vi "MultiTrigBurst.vi"(2 "high time":dbl=1e-05 format="%^.2e", 3 "Digitizer Settings":T1={"Digitizer delay (us) "=0.0, "rf points per line"=2048, "lines per plane"=128, "Samp Rate (Hz)"=100000000.0, "Additional dig delay (us)"=0.0, "Voltage Scale"=0.4, "Pre-Looks"=0, "Offset delay (us)"=0.0, "bits A/D"=8, "Avg Num"=1, "DigTimeOut"=5.0, "Rel Dig Delay"=0.0, "Dig Ch"=0, "LeCroyCluster"={"LeCroy Channels"=[TRUE, FALSE, FALSE, FALSE], "LC read pt offset"=0.0, "Sweep Avg"=FALSE}, "Main Digitizer"=enum."NI Digitizer", "Dig Config"=enum."Single channel", "Digitizer ID Cluster"={"Acqiris/Alazar/SP ID"=[], "NI Instr Handles"=[], "LeCroy VISA"="", "GaGe Handle"={"Handle"=0, "Sample size"=0, "Resolution"=0, "Offset"=0, "Channels"=0, "Boards"=0}, "ATS Ref"="ATS9350", "Acqiris Address"=["PCI::INSTR0"], "ADQRef"=refnum, "adq_cu_ptr"=refnum}, "Trigger Settings"={"Trig Source"=1, "Trig Coupling"=0, "Trig Slope"=0, "Level (mV)"=1500.0}, "Bulk Acq"=FALSE, "Bulk Start Indexes"=[], "Data Ref RF"=refnum, "NI ID/Channel"=[], "Total Dig CH"=1, "Xtra Ann Trig delay (us)"=10.0, "Fix Z Delay?"=FALSE, "One Way Transmission?"=FALSE, "Data Ref Log"=refnum} {"Trigger Settings"."Trig Slope" items=["Positive", "Negative"]; "Trigger Settings"."Level (mV)" format="%.2f"; "Trigger Settings"."Trig Coupling" items=["DC 1 MOhm", "AC 1 MOhm", "DC 50 Ohm", "AC 50 Ohm"]; "Trigger Settings"."Trig Source" items=["Chan 1", "External"]; "Rel Dig Delay" format="%.2f"; "DigTimeOut" format="%.2f"; "Avg Num" min=1; "Offset delay (us)" format="%.2f"; "Additional dig delay (us)" format="%.2f"; "Digitizer delay (us)" format="%.2f"}, 4 "error in":errorcluster, 5 "Output Pulse#":i32=2, 6 "Counter(s)":tag="Dev1/ctr1", 7 "Source":tag="/Dev1/PFI9" caption="Trigger Source") -> (0 "error out":errorcluster, 1 "task out":refnum<k21>)   [LabVIEW 2022 SP3]
uses:
  Digitizers/-DigitizerRoutines/DigitizerSettings.ctl
  Digitizers/-DigitizerRoutines/Digitizer.ctl
  Digitizers/-DigitizerRoutines/DigConfig.ctl
  Digitizers/-DigitizerRoutines/DigitizerID.ctl
  C:/Windows/System32/ADQAPI_dotNet_helper.dll
  Motion Controllers/-MotionRoutines/MotionGlobals.vi
  Switch Modules/SwitchGlobals.vi
  <vilib>/DAQmx/create/channels.llb/DAQmx Create Channel (CO-Pulse Generation-Time).vi
  <vilib>/DAQmx/configure/timing.llb/DAQmx Timing (Implicit).vi
  <vilib>/DAQmx/configure/trigger.llb/DAQmx Start Trigger (Digital Edge).vi
  <resource>/objmgr/daqmx.rc
panel:
  in  "Trigger Edge":i32(ring)=10280 items=["Rising"=10280, "Falling"=10171]
  # "Counter 1 output is the BNC on grey box."
  # "Trigger source comes from Gate of CTR0 (PFI9)\n\nThe NI trigger connector routes to CTR0 Gate\n\nConnect Ther Ext Trigger to digitizer\n\nNeed to turn global variable on for Retro pulse\n\nUse delay and window pluse high time to determine interval between"
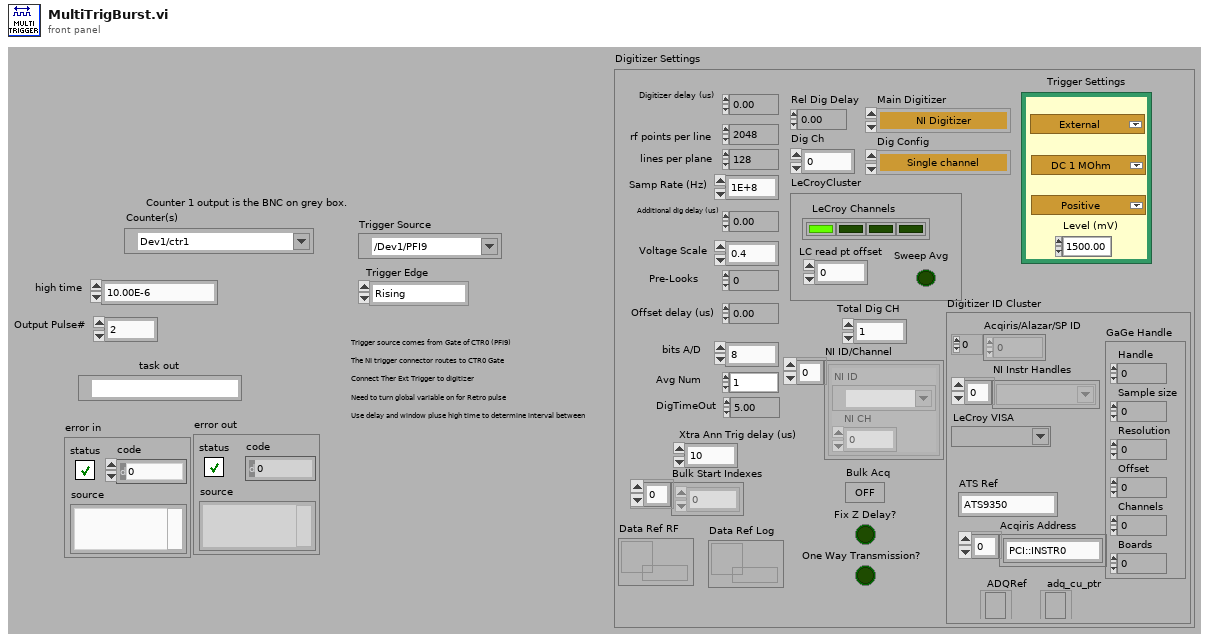
[diagram p1: front panel]
types:
  T1 = typedef "DigitizerSettings.ctl" = cluster{"Digitizer delay (us) ":dbl, "rf points per line":i32, "lines per plane":i32, "Samp Rate (Hz)":dbl, "Additional dig delay (us)":dbl, "Voltage Scale":dbl, "Pre-Looks":i32, "Offset delay (us)":dbl, "bits A/D":i8, "Avg Num":i32, "DigTimeOut":sgl, "Rel Dig Delay":sgl, "Dig Ch":i32, "LeCroyCluster":cluster{"LeCroy Channels":bool[], "LC read pt offset":dbl, "Sweep Avg":bool}, "Main Digitizer":T2, "Dig Config":T3, "Digitizer ID Cluster":T4, "Trigger Settings":cluster{"Trig Source":u16, "Trig Coupling":u16, "Trig Slope":u16, "Level (mV)":dbl}, "Bulk Acq":bool, "Bulk Start Indexes":i32[], "Data Ref RF":refnum<data-value>, "NI ID/Channel":cluster{"NI ID":refnum<k15>, "NI CH":i32}[], "Total Dig CH":i32, "Xtra Ann Trig delay (us)":dbl, "Fix Z Delay?":bool, "One Way Transmission?":bool, "Data Ref Log":refnum<data-value>}
  T2 = typedef "Digitizer.ctl" = enum16{"Acqiris Digitizer", "NI Digitizer", "LeCroy", "GaGe", "AlazarTech", "No Digitizer", "Teledyne"}
  T3 = typedef "DigConfig.ctl" = enum16{"Single channel", "2 Chans w/ 2 Acqiris", "2 Chans w/ 1 Acqiris", "5-CH Pulser New", "5-CH pulser w/ ann array", "5-pass style ann array", "Empty"}
  T4 = typedef "DigitizerID.ctl" = cluster{"Acqiris/Alazar/SP ID":u32[], "NI Instr Handles":refnum<k15>[], "LeCroy VISA":refnum<visa-resource-name>, "GaGe Handle":cluster{"Handle":u32, "Sample size":u32, "Resolution":i32, "Offset":i32, "Channels":u32, "Boards":u32}, "ATS Ref":string, "Acqiris Address":string[], "ADQRef":refnum<k24>, "adq_cu_ptr":refnum<k24>}
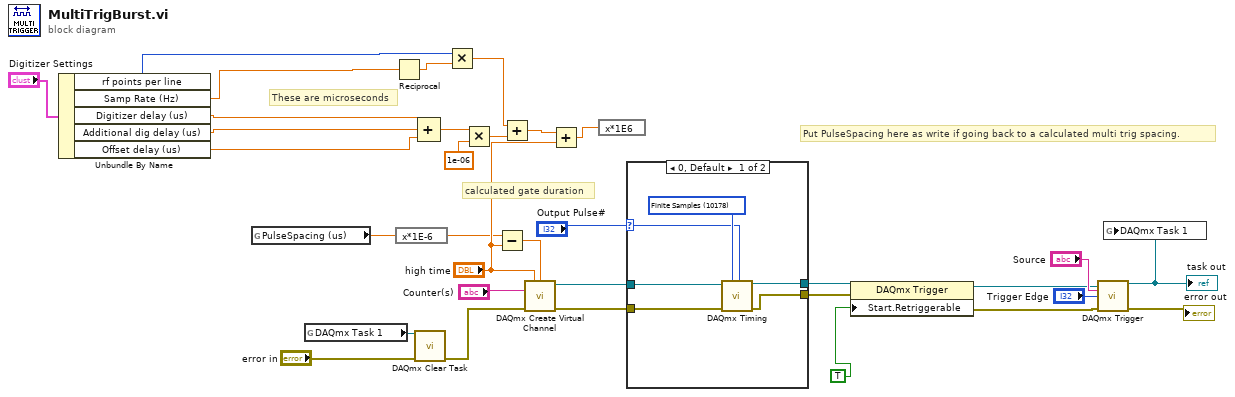
[diagram p0: block diagram]
diagram:
  # "Put PulseSpacing here as write if going back to a calculated multi trig spacing."
  # "calculated gate duration"
  # "These are microseconds"
  n1 = Unbundle By Name("Digitizer Settings") -> ("rf points per line"=w6:i32, "Samp Rate (Hz)"=w7:dbl, "Digitizer delay (us)"=w5:dbl, "Additional dig delay (us)"=w4:dbl, "Offset delay (us)"=w3:dbl)
  n2 = global read "SwitchGlobals.vi" "PulseSpacing (us)"() -> (w1:sgl)
  n3 = global read "MotionGlobals.vi" "DAQmx Task 1"() -> (w16:refnum<k21>)
  n4 = Reciprocal(x=w7) -> (1/x=w18:dbl)
  n5 = expression code="x*1E-6"(w1) -> (w10:sgl)
  n6 = call <vilib>:"DAQmx Clear Task.vi"("task in"=w16, "error in"="error in") -> ("error out"=w15:errorcluster)  [unwired: 13 out]
  n7 = Compound Arithmetic op=ADD(w5, w4, w3) -> (w27:dbl)
  n8 = Multiply(x=w6, y=w18) -> (x*y=w25:dbl)
  n9 = Multiply(x=w27, y=1e-06) -> (x*y=w24:dbl)
  n10 = Subtract(x=w10, y="high time") -> (x-y=w11:dbl)
  n11 = Add(x=w25, y=w24) -> (x+y=w12:dbl)
  n12 = call-poly <vilib>:"DAQmx Create Virtual Channel.vi"("high time"="high time", "low time"=w11, "counter"="Counter(s)", "error in"=w15) -> ("task out"=w32:refnum<k21>, "error out"=w33:errorcluster)  [unwired: 5 in, 5 out]
  n13 = Add(x=w12, y="high time") -> (x+y=w14:dbl)
  n14 = expression code="x*1E6"(w14) -> ()  [unwired: 1 out]
  n15 = case shown="0, Default" "Output Pulse#" {
    selector: "Output Pulse#" -> [w34 _]
    tunnel: w33 -> [w39 w40]
    tunnel: w32 -> [w38 w41]
    tunnel: [w36 w41] -> w23
    tunnel: [w35 w40] -> w22
    frame 0, Default {
      w37 = 10178 items=["Finite Samples"=10178, "Continuous Samples"=10123] ("sample mode")
      n16 = call-poly <vilib>:"DAQmx Timing.vi"("task/channels in"=w38, "sample mode"=w37, "samples per channel"=w34, "error in"=w39) -> ("task out"=w36:refnum<k21>, "error out"=w35:errorcluster)  [unwired: 2 in, 8 out]
    }
    frame 1 {
    }
  }
  n17 = property class="DAQmx Trigger"(reference=w23, error in=w22, "Start.Retriggerable"=TRUE) -> (reference out=w21:refnum<k21>, error out=w20:errorcluster)
  n18 = call-poly <vilib>:"DAQmx Trigger.vi"("task/channels in"=w21, "source"="Source", "edge"="Trigger Edge", "error in"=w20) -> ("task out"=w28:refnum<k21>, "error out"=→"error out":errorcluster)  [unwired: 10 out]
  "task out" <- w28
  n19 = global write "MotionGlobals.vi" "DAQmx Task 1"(w28) -> ()
